vi "EnterPassword.vi"(6 "Message":string="Press OK to Enter Password or Cancel to Quit ", 8 "error in (no error)":errorcluster, 11 "Enable(t)":bool) -> (0 "error out":errorcluster, 3 "success(t)":bool, 5 "cancelled(t)":bool)   [LabVIEW 2018]
uses:
  Initialize References/Sequence Globals.vi
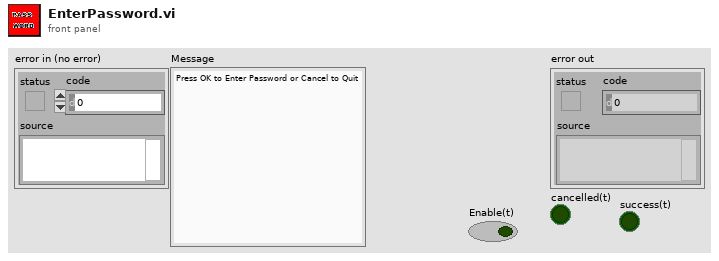
[diagram p1: front panel]
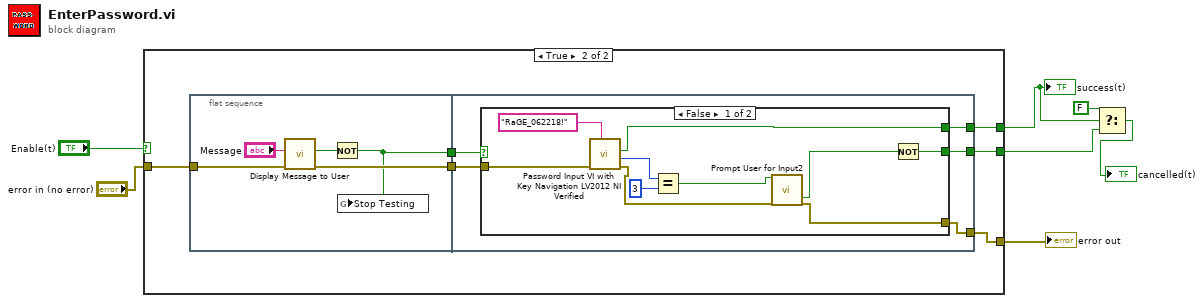
[diagram p0: block diagram]
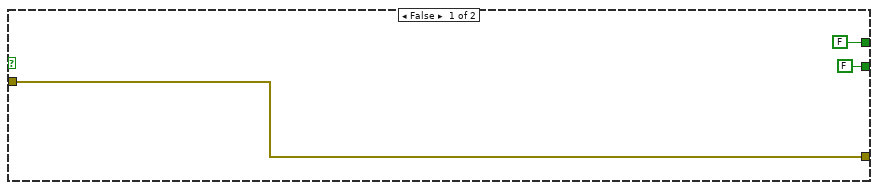
[diagram p2: hidden frame]
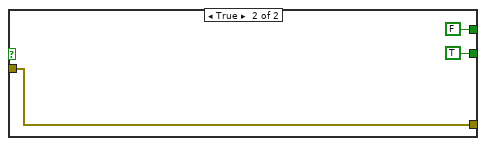
[diagram p3: hidden frame]
diagram:
  n1 = case shown="True" "Enable(t)" {
    tunnel: "error in (no error)" -> [w10 w16]
    tunnel: [w10 w13] -> w5
    tunnel: [FALSE ("Password Correct?") w15] -> w4
    tunnel: [FALSE w12] -> w1
    frame False {
    }
    frame True {
      n2 = flat-sequence {
        tunnel: w16 -> [w20]
        tunnel: [w21] -> w14
        tunnel: [w17] -> w11
        tunnel: [w26] -> w15
        tunnel: [w25] -> w13
        tunnel: [w24] -> w12
        tunnel: w14 -> [w23]
        tunnel: w11 -> [w22]
        frame #0 {
          n3 = call "Display Message to User"("error in (no error)"=w20, "Message"="Message") -> ("error out"=w21:errorcluster, "OK"=w19:bool)  [unwired: 8 in]
          n4 = Not(x=w19) -> (.not. x?=w17:bool)
          n5 = global write "Sequence Globals.vi" "Stop Testing"(w17) -> ()
        }
        frame #1 {
          n6 = case shown="False" w22 {
            tunnel: [w35 FALSE ("Password Correct?")] -> w26
            tunnel: [w33 w37] -> w25
            tunnel: [w31 TRUE] -> w24
            tunnel: w23 -> [w27 w37]
            frame False {
              n7 = call "Password Input VI with Key Navigation LV2012 NI Verified.vi"("The Password"="RaGE_062218!", "error in (no error)"=w27) -> ("error out"=w34:errorcluster, "Number of Incorrect Responses"=w29:i32, "Password Correct?"=w35:bool)  [unwired: 7 in]
              n8 = Equal?(x=w29, y=3) -> (x = y?=w36:bool)
              n9 = call "Prompt User for Input2"("Enable"=w36, "error in (no error)"=w34) -> ("OK"=w32:bool, "error out"=w33:errorcluster)  [unwired: 16 in]
              n10 = Not(x=w32) -> (.not. x?=w31:bool)
            }
            frame True {
            }
          }
        }
      }
    }
  }
  "error out" <- w5
  "success(t)" <- w4
  n11 = Select(t=FALSE, s=w4, f=w1) -> (s? t:f=→"cancelled(t)":bool)
